vi "EXO_DB_Write.vi"() -> ()   [LabVIEW 2012]
uses:
  <vilib>/addons/database/NI_Database_API.lvlib
  <vilib>/addons/database/Connection.llb/DB Tools Open Connec (Path).vi
panel:
  in  "V-15":bool
  in  "V-14":bool
  in  "V-13":bool
  in  "V-12":bool
  in  "V-11":bool
  in  "V-10":bool
  in  "V-9":bool
  in  "V-8":bool
  in  "V-7":bool
  in  "V-6":bool
  in  "V-5":bool
  in  "V-4":bool
  in  "V-3":bool
  in  "V-2":bool
  in  "V-1":bool
  in  "Flow Speed":dbl
  in  "Pressure 3":dbl
  in  "Pressure 2":dbl
  in  "Pressure 1":dbl
  in  "LN2 Level_Dewar 2":dbl
  in  "LN2 Level_Dewar 1":dbl
  in  "Xe Level":dbl
  in  "Temperature 3_Thermocouple":dbl
  in  "Temperature 2_DT":dbl
  in  "Temperature 1_PT":dbl
  in  "stop":bool
  in  "Table Name (The table that you want to save the data into)":string="EXO"
  # "EXO DatabaseWrite Sub-VI"
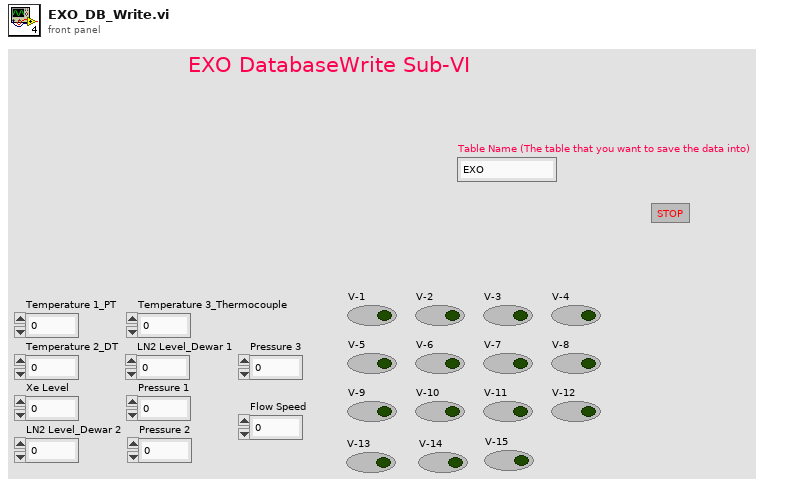
[diagram p1: front panel]
types:
  T1 = typedef "NI_Database_API.lvlib/Conn ObjectReference.ctl" = refnum<k1>
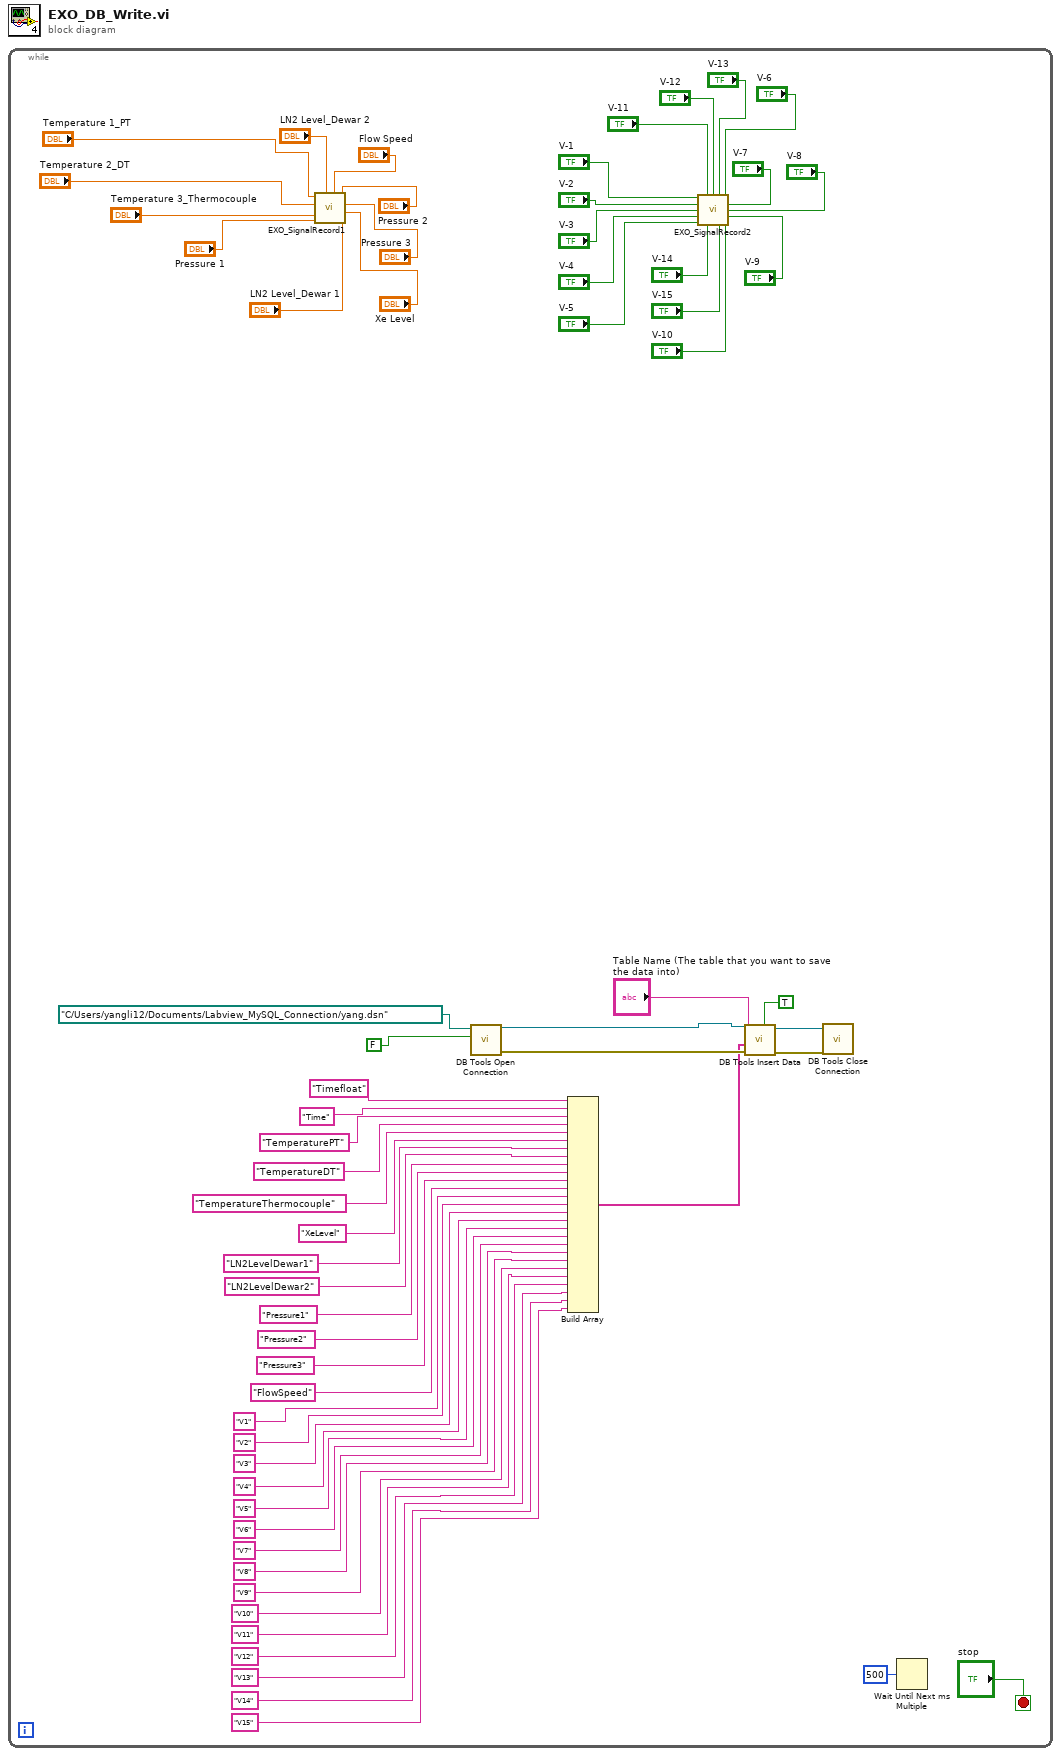
[diagram p0: block diagram]
diagram:
  n1 = while {
    stop <- "stop" stop-if-true
    n2 = call "EXO_SignalRecord1.vi"("LN2 Level_Dewar 1"="LN2 Level_Dewar 1", "Xe Level"="Xe Level", "Pressure 3"="Pressure 3", "Pressure 2"="Pressure 2", "Flow Speed"="Flow Speed", "LN2 Level_Dewar 2"="LN2 Level_Dewar 2", "Pressure 1"="Pressure 1", "Temperature 3_Thermocouple"="Temperature 3_Thermocouple", "Temperature 2_DT"="Temperature 2_DT", "Temperature 1_PT"="Temperature 1_PT") -> ()  [unwired: 1 in, 1 out]
    n3 = call-poly <vilib>:"DB Tools Open Connection.vi"("prompt? (F)"=FALSE, "connection information"=path "C:/Users/yangli12/Documents/Labview_MySQL_Connection/yang.dsn") -> ("error out"=w59:errorcluster, "connection reference"=w60:T1)  [unwired: 6 in]
    n4 = Build Array("Timefloat" ("element"), "Time" ("table"), "TemperaturePT" ("table"), "TemperatureDT" ("table"), "TemperatureThermocouple" ("table"), "XeLevel" ("table"), "LN2LevelDewar1" ("table"), "LN2LevelDewar2" ("table"), "Pressure1" ("table"), "Pressure2" ("table"), "Pressure3" ("table"), "FlowSpeed" ("table"), "V1" ("table"), "V2" ("table"), "V3" ("table"), "V4" ("table"), "V5" ("table"), "V6" ("table"), "V7" ("table"), "V8" ("table"), "V9" ("table"), "V10" ("table"), "V11" ("table"), "V12" ("table"), "V13" ("table"), "V14" ("table"), "V15" ("table")) -> (w55:string[])
    n5 = call "EXO_SignalRecord2.vi"("V-1"="V-1", "V-11"="V-11", "V-12"="V-12", "V-13"="V-13", "V-6"="V-6", "V-2"="V-2", "V-7"="V-7", "V-3"="V-3", "V-8"="V-8", "V-4"="V-4", "V-9"="V-9", "V-5"="V-5", "V-14"="V-14", "V-15"="V-15", "V-10"="V-10") -> ()  [unwired: 1 out]
    n6 = call <vilib>:"DB Tools Insert Data.vi"("create table? (F)"=TRUE, "error in (no error)"=w59, "columns"=w55, "table"="Table Name (The table that you want to save the data into)", "connection reference"=w60) -> ("error out"=w52:errorcluster, "connection reference out"=w53:T1)  [unwired: 5 in]
    n7 = call <vilib>:"DB Tools Close Connection.vi"("error in (no error)"=w52, "connection reference"=w53) -> ()  [unwired: 5 in, 1 out]
    n8 = Wait Until Next ms Multiple(millisecond multiple=u32 500) -> ()  [unwired: 1 out]
  }
